vi "ellipsetest.vi"() -> ()   [LabVIEW 2013]
uses:
  <vilib>/measure/NI_MABase.lvlib
panel:
  out "Waveform Graph 4":dbl[](graph)
  out "Waveform Graph 3":dbl[](graph)
  out "ox":dbl
  out "oy":dbl
  out "x":dbl
  out "y":dbl
  out "max index(es)":i32
  out "S":dbl
  out "L":dbl
  out "phi":dbl
  out "Xc":dbl
  out "Yc":dbl
  out "Waveform Graph 2":dbl[](graph)
  out "Waveform Graph":dbl[][](graph)
  out "Intensity Graph":dbl[][](graph)
  in  "angle":dbl format="%#_13g"
  out "XY Graph":cluster{dbl[], dbl[]}[](graph)
  out "Angle ref":dbl
  out "Vy-min ref":dbl=-9.0
  out "Vy-max ref":dbl=9.0
  out "Vx-min ref":dbl=-9.0
  out "Vx-max ref":dbl=9.0
  out "xpixels ref":i32=256 caption="x-res"
  out "ypixels ref":i32=256 caption="y-res]"
  in  "avpp":i32=1 caption="# averages\n per point" min=1 step=1
  in  "phase 2":dbl format="%.2p"
  in  "phase":dbl format="%.2p"
  in  "Sampling rate":dbl=400000.0 min=1.0 step=1.0
  out "ROI Type":u16(ring) items=["Rectangle", "Circle", "Freeform Boundary", "Freeform Interior"]
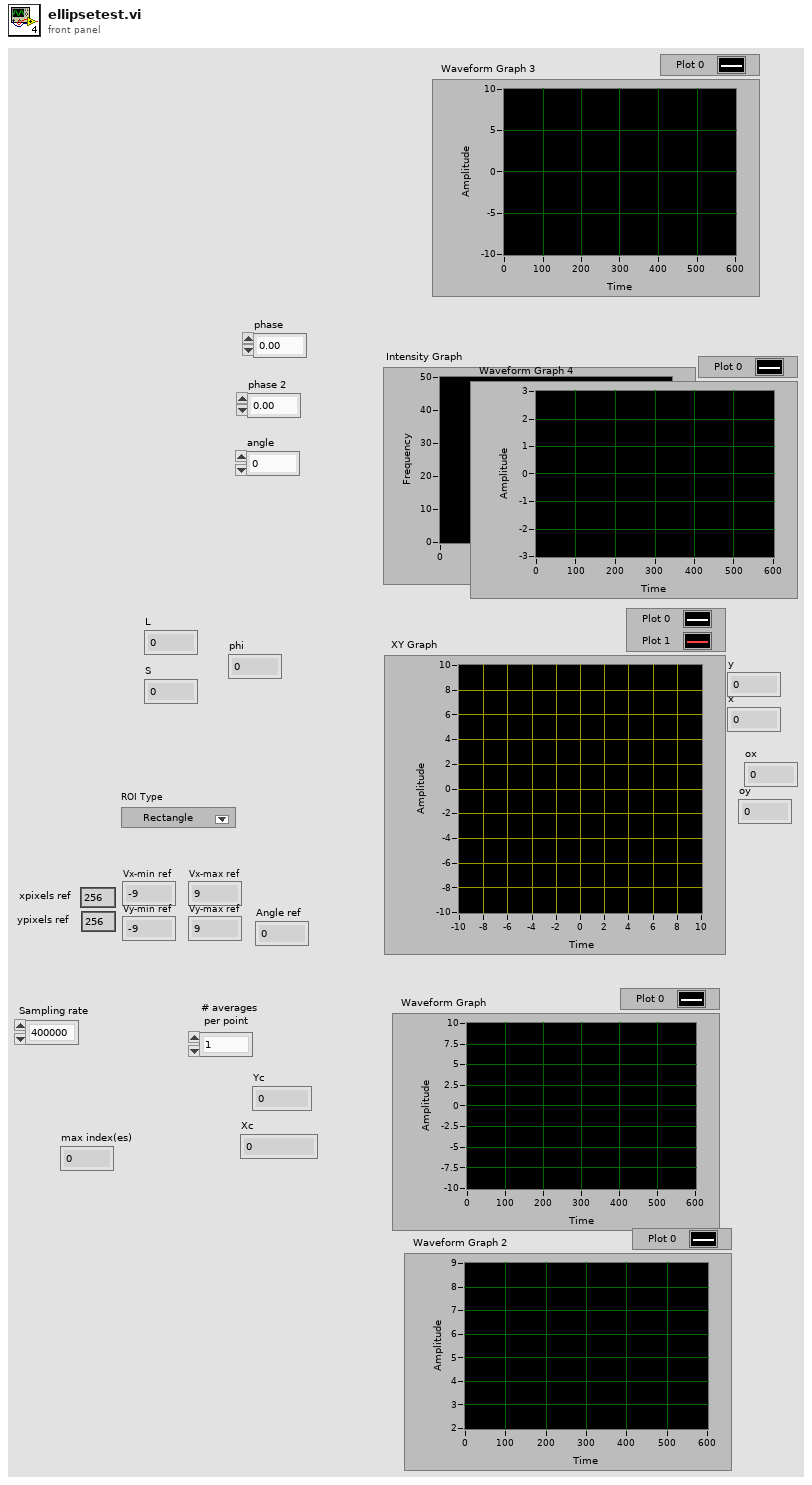
[diagram p1: front panel]
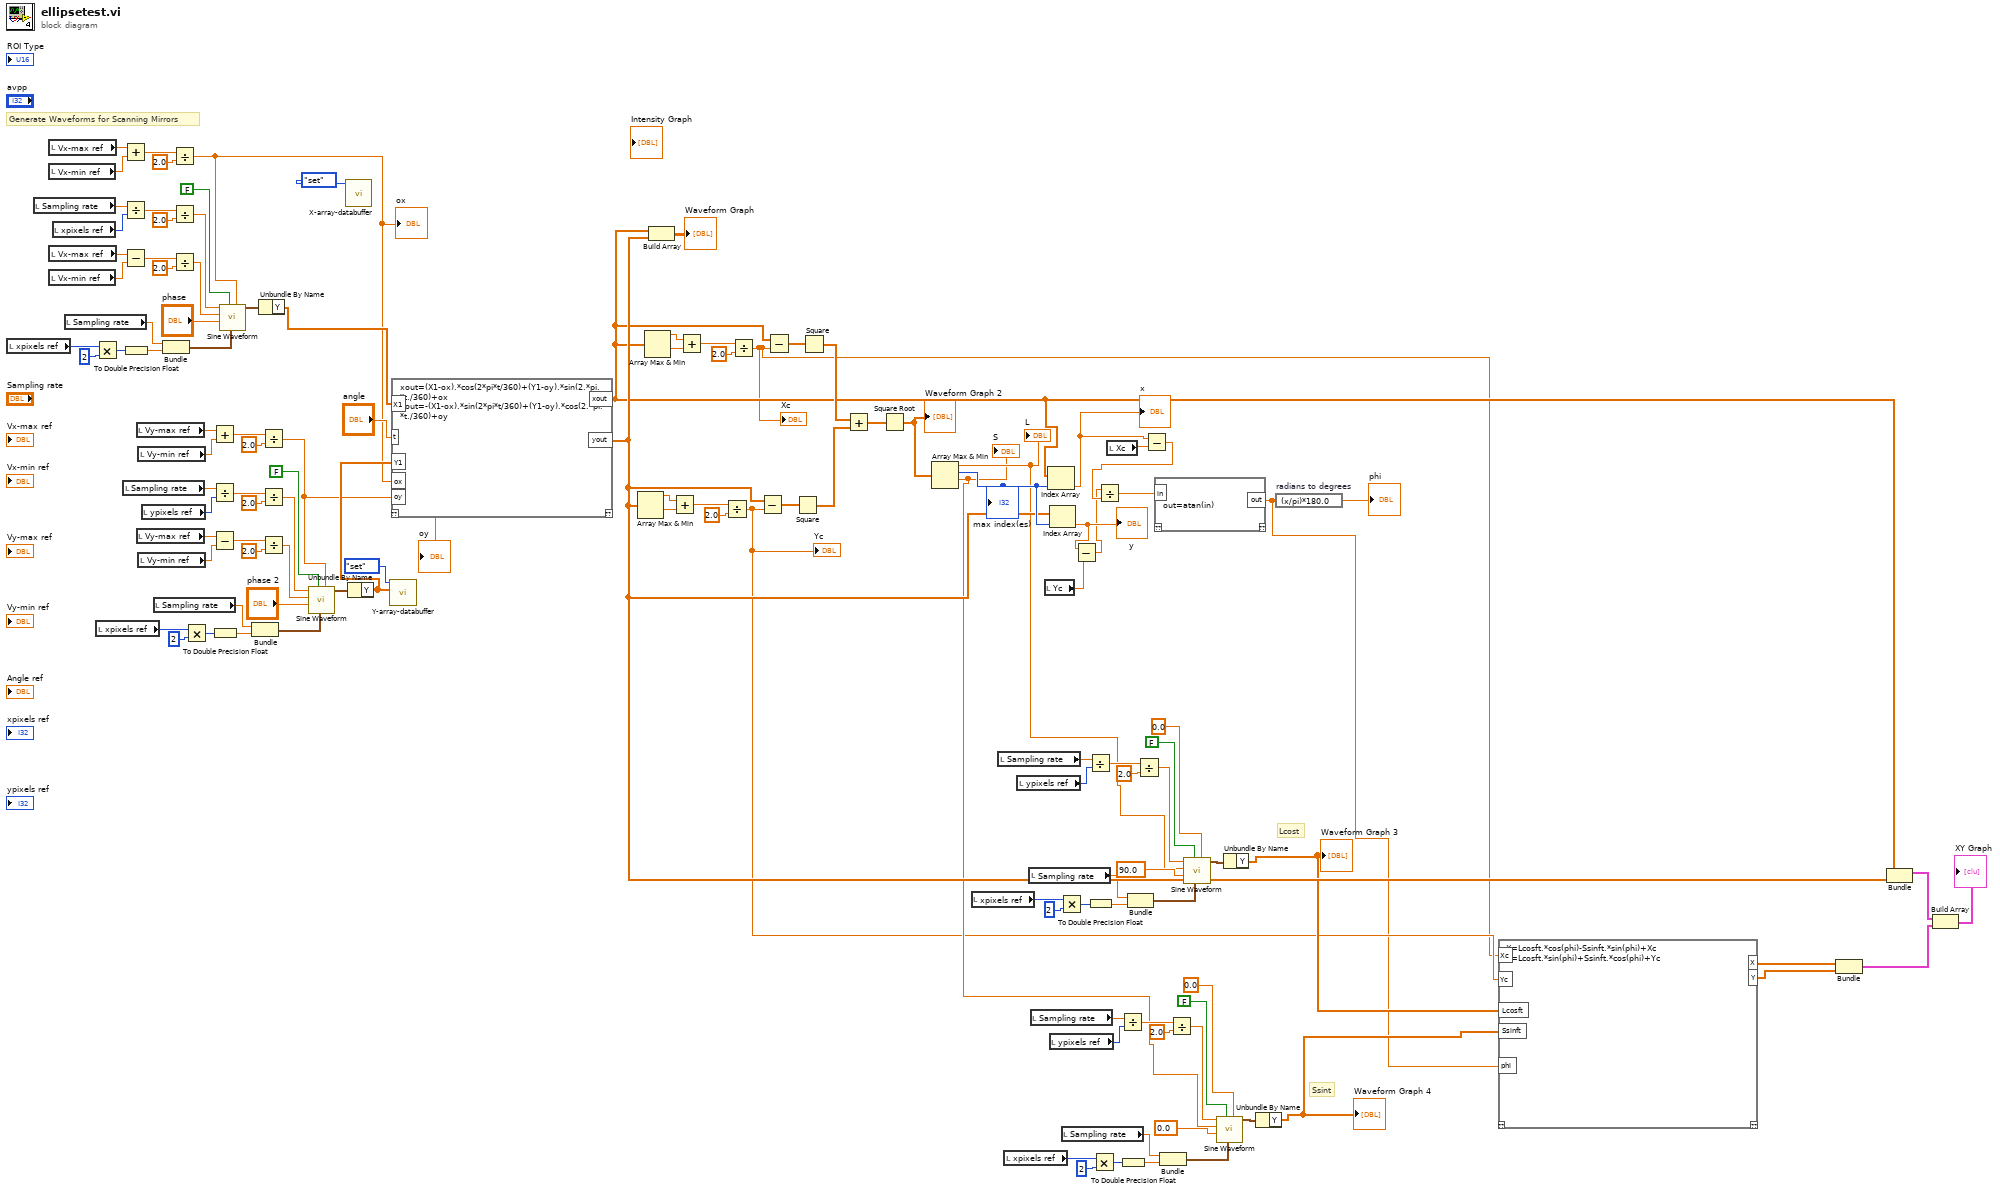
[diagram p0: block diagram]
diagram:
  # "Ssint"
  # "Lcost"
  # "Generate Waveforms for Scanning Mirrors"
  n1 = local read "xpixels ref"() -> (w108:i32)
  n2 = local read "Sampling rate"() -> (w97:dbl)
  n3 = local read "Vx-max ref"() -> (w101:dbl)
  n4 = local read "Vx-min ref"() -> (w102:dbl)
  n5 = local read "Vx-max ref"() -> (w114:dbl)
  n6 = local read "Vx-min ref"() -> (w113:dbl)
  n7 = local read "xpixels ref"() -> (w119:i32)
  n8 = local read "Sampling rate"() -> (w109:dbl)
  n9 = Multiply(x=w108, y=2) -> (x*y=w106:i32)
  n10 = local read "xpixels ref"() -> (w85:i32)
  n11 = Add(x=w101, y=w102) -> (x+y=w99:dbl)
  n12 = Divide(x=w97, y=w119) -> (x/y=w118:dbl)
  n13 = Subtract(x=w114, y=w113) -> (x-y=w112:dbl)
  n14 = local read "Sampling rate"() -> (w96:dbl)
  n15 = To Double Precision Float(number=w106) -> (double precision float=w104:dbl)
  n16 = local read "Vy-max ref"() -> (w92:dbl)
  n17 = local read "Vy-max ref"() -> (w80:dbl)
  n18 = local read "Vy-min ref"() -> (w91:dbl)
  n19 = local read "Vy-min ref"() -> (w81:dbl)
  n20 = local read "ypixels ref"() -> (w75:i32)
  n21 = local read "Sampling rate"() -> (w84:dbl)
  n22 = Bundle("Sampling rate"=w109, w104) -> (w105:cluster{"Sampling rate":dbl, dbl})  [unwired: 1 in]
  n23 = Divide(x=w99, y=2.0) -> (x/y=w61:dbl)
  "ox" <- w61
  n24 = Divide(x=w118, y=2.0) -> (x/y=w116:dbl)
  n25 = Divide(x=w112, y=2.0) -> (x/y=w111:dbl)
  n26 = Multiply(x=w85, y=2) -> (x*y=w87:i32)
  n27 = Add(x=w92, y=w91) -> (x+y=w94:dbl)
  n28 = Divide(x=w96, y=w75) -> (x/y=w76:dbl)
  n29 = Subtract(x=w80, y=w81) -> (x-y=w82:dbl)
  n30 = To Double Precision Float(number=w87) -> (double precision float=w89:dbl)
  n31 = call <vilib>:"Sine Waveform.vi"("offset"=w61, "sampling info"=w105, "reset signal"=FALSE, "phase"="phase", "amplitude"=w111, "frequency"=w116) -> ("signal out"=w98:waveform(dbl))  [unwired: 4 in, 1 out]
  n32 = Bundle("Sampling rate"=w84, w89) -> (w88:cluster{"Sampling rate":dbl, dbl})  [unwired: 1 in]
  n33 = Unbundle By Name(w98) -> ("Y"=w72:dbl[])
  n34 = Divide(x=w94, y=2.0) -> (x/y=w62:dbl)
  "oy" <- w62
  n35 = Divide(x=w76, y=2.0) -> (x/y=w78:dbl)
  n36 = Divide(x=w82, y=2.0) -> (x/y=w74:dbl)
  n37 = call <vilib>:"Sine Waveform.vi"("offset"=w62, "sampling info"=w88, "reset signal"=FALSE, "phase"="phase 2", "amplitude"=w74, "frequency"=w78) -> ("signal out"=w95:waveform(dbl))  [unwired: 4 in, 1 out]
  n38 = call "X-array-databuffer.vi"("command"=enum16{"get", "set", "clear", "append"}."set") -> ()  [unwired: 3 in, 2 out]
  n39 = Unbundle By Name(w95) -> ("Y"=w73:dbl[])
  n40 = call "Y-array-databuffer.vi"("array in"=w73, "command"=enum16{"get", "set", "clear", "append"}."set") -> ()  [unwired: 2 in, 2 out]
  n41 = script code="xout=(X1-ox).*cos(2*pi*t/360)+(Y1-oy).*sin(2.*pi.*t./360)+ox\nyout=-(X1-ox).*sin(2*pi*t/360)+(Y1-oy).*cos(2.*pi.*t./360)+oy"("X1"=w72, "Y1"=w73, "t"="angle", "ox"=w61, "oy"=w62) -> ("xout"=w51:dbl[], "yout"=w52:dbl[])  [unwired: 1 in, 1 out]
  n42 = Array Max & Min(array=w52) -> (max value=w65:dbl, min value=w58:dbl)  [unwired: 2 out]
  n43 = Array Max & Min(array=w51) -> (max value=w57:dbl, min value=w56:dbl)  [unwired: 2 out]
  n44 = Build Array(w51, w52) -> (→"Waveform Graph":dbl[][])
  n45 = Add(x=w65, y=w58) -> (x+y=w67:dbl)
  n46 = Add(x=w57, y=w56) -> (x+y=w69:dbl)
  n47 = Divide(x=w67, y=2.0) -> (x/y=w9:dbl)
  "Yc" <- w9
  n48 = Divide(x=w69, y=2.0) -> (x/y=w8:dbl)
  "Xc" <- w8
  n49 = Subtract(x=w52, y=w9) -> (x-y=w64:dbl[])
  n50 = Subtract(x=w51, y=w8) -> (x-y=w63:dbl[])
  n51 = Square(x=w64) -> (x^2=w53:dbl[])
  n52 = Square(x=w63) -> (x^2=w54:dbl[])
  n53 = Add(x=w54, y=w53) -> (x+y=w60:dbl[])
  n54 = Square Root(x=w60) -> (sqrt(x)=w59:dbl[])
  "Waveform Graph 2" <- w59
  n55 = Array Max & Min(array=w59) -> (max value=w28:dbl, max index (indices)=w55:i32, min value=w12:dbl)  [unwired: 1 out]
  "L" <- w28
  "S" <- w12
  "max index(es)" <- w55
  n56 = local read "xpixels ref"() -> (w37:i32)
  n57 = local read "Sampling rate"() -> (w31:dbl)
  n58 = local read "xpixels ref"() -> (w19:i32)
  n59 = local read "ypixels ref"() -> (w43:i32)
  n60 = local read "Sampling rate"() -> (w38:dbl)
  n61 = local read "Sampling rate"() -> (w25:dbl)
  n62 = local read "Yc"() -> (w46:dbl)
  n63 = Index Array(array=w51, index=w55) -> (element=w49:dbl)
  "x" <- w49
  n64 = Index Array(array=w52, index=w55) -> (element=w45:dbl)
  "y" <- w45
  n65 = local read "ypixels ref"() -> (w13:i32)
  n66 = Multiply(x=w37, y=2) -> (x*y=w35:i32)
  n67 = local read "Sampling rate"() -> (w18:dbl)
  n68 = Subtract(x=w45, y=w46) -> (x-y=w44:dbl)
  n69 = Divide(x=w31, y=w43) -> (x/y=w42:dbl)
  n70 = To Double Precision Float(number=w35) -> (double precision float=w33:dbl)
  n71 = Multiply(x=w19, y=2) -> (x*y=w21:i32)
  n72 = local read "Xc"() -> (w47:dbl)
  n73 = Divide(x=w25, y=w13) -> (x/y=w14:dbl)
  n74 = To Double Precision Float(number=w21) -> (double precision float=w23:dbl)
  n75 = Bundle("Sampling rate"=w38, w33) -> (w34:cluster{"Sampling rate":dbl, dbl})  [unwired: 1 in]
  n76 = Divide(x=w42, y=2.0) -> (x/y=w40:dbl)
  n77 = Subtract(x=w49, y=w47) -> (x-y=w48:dbl)
  n78 = Divide(x=w44, y=w48) -> (x/y=w50:dbl)
  n79 = script code="out=atan(in)"("in"=w50) -> ("out"=w2:dbl)  [unwired: 1 in, 1 out]
  n80 = Bundle("Sampling rate"=w18, w23) -> (w22:cluster{"Sampling rate":dbl, dbl})  [unwired: 1 in]
  n81 = Divide(x=w14, y=2.0) -> (x/y=w16:dbl)
  n82 = call <vilib>:"Sine Waveform.vi"("offset"=0.0, "sampling info"=w34, "reset signal"=FALSE, "phase"=90.0 ("phase 3"), "amplitude"=w28, "frequency"=w40) -> ("signal out"=w29:waveform(dbl))  [unwired: 4 in, 1 out]
  n83 = call <vilib>:"Sine Waveform.vi"("offset"=0.0, "sampling info"=w22, "reset signal"=FALSE, "phase"=0.0 ("phase 3"), "amplitude"=w12, "frequency"=w16) -> ("signal out"=w27:waveform(dbl))  [unwired: 4 in, 1 out]
  n84 = Unbundle By Name(w29) -> ("Y"=w11:dbl[])
  "Waveform Graph 3" <- w11
  n85 = Unbundle By Name(w27) -> ("Y"=w10:dbl[])
  "Waveform Graph 4" <- w10
  n86 = expression code="(x/pi)*180.0" "radians to degrees"(w2) -> (→"phi":dbl)
  n87 = script code="X=Lcosft.*cos(phi)-Ssinft.*sin(phi)+Xc\nY=Lcosft.*sin(phi)+Ssinft.*cos(phi)+Yc"("Xc"=w8, "Yc"=w9, "Lcosft"=w11, "Ssinft"=w10, "phi"=w2) -> ("X"=w7:dbl[], "Y"=w6:dbl[])  [unwired: 1 in, 1 out]
  n88 = Bundle(w7, w6) -> (w5:cluster{dbl[], dbl[]})  [unwired: 1 in]
  n89 = Bundle(w51, w52) -> (w4:cluster{dbl[], dbl[]})  [unwired: 1 in]
  n90 = Build Array(w4, w5) -> (→"XY Graph":cluster{dbl[], dbl[]}[])
